vi "Get Channel Array Offset.vi"(0 "private data":T1={"instruction target"=refnum, "channels"=[], "measure state"=enum."Uninitialized", "rx output divider"=enum."1", "equalization mode"=enum."DFE", "rx internal data width"=enum."32 Bit", "BER floor"=0.0, "number of points completed"=0, "rx output divider configured?"=FALSE, "equalization mode configured?"=FALSE, "rx data width configured?"=FALSE}, 5 "instance":u8, 11 "error in":errorcluster) -> (4 "private data out":T1={"instruction target"=refnum, "channels"=[], "measure state"=enum."Uninitialized", "rx output divider"=enum."1", "equalization mode"=enum."DFE", "rx internal data width"=enum."32 Bit", "BER floor"=0.0, "number of points completed"=0, "rx output divider configured?"=FALSE, "equalization mode configured?"=FALSE, "rx data width configured?"=FALSE}, 6 "channel array offset":i32, 15 "error out":errorcluster)   [LabVIEW 2015, in "niHighSpeedSerial Eye Scan v1 Host.lvclass"]
doc: "Returns the offset in the channels array of the specified instance number\n\n<B>Input Parameters</B>\n\n<B>private data</B> is the class private data input into the VI.\n\n<B>private data.instruction target</B> is the instruction target to use when communicating with the FPGA.\n\n<B>private data.channels</B> is the array of channel information.\n\n<B>private data.channels.instance</B> is the instance of the channel.\n\n<B>private data.channels.channel</B> is the channel object for a particular channel instance.\n\n<B>private data.channels.point iterator</B> is the point iterator which stores the channel's measured points and controls which point to measure next.\n\n<B>private data.measure state</B> maintains the internal state of the Eye Scan class.\nenum values: Uninitialized,Initialized,Ready,Measuring,Finished,Aborted\n\n<B>private data.rx output divider</B> represents the configuration of the receiver output divider. This should match the values configured with RXRATE and RXOUT_DIV.\nenum values: 1,2,4,8,16\n\n<B>private data.equalization mode</B> indicates the Equalization Mode that the lane is using.\nenum values: DFE,LPM\n\n<B>private data.data width</B> is the data width (in bits) of the receiver lane.\nenum values: 16 Bit,20 Bit,32 Bit,40 Bit\n\n<B>private data.BER floor</B> is the minimum Bit Error Rate which may be computed.\n\n<B>private data.number of points completed</B> is the number of points that have been completed so far by Eye Scan.\n\n<B>private data.rx output divider configured?</B> is true if you have configured the RX Output Divider.\n\n<B>private data.equalization mode configured?</B> is true if you have configured the Equalization Mode\n\n<B>private data.data width configured?</B> is true if you have configured the Data Width.\n\n<B>instance</B> The instance of the channel to be used.\n\n<B>error in</B> describes error conditions that occur before this node runs. This input provides standard 'error in' functionality.\n\n<B>Output Parameters</B>\n\n<B>private data out</B> is the class private data output from the VI.\n\n<B>private data out.instruction target</B> is the instruction target to use when communicating with the FPGA.\n\n<B>private data out.channels</B> is the array of channel information.\n\n<B>private data out.channels.instance</B> is the instance of the channel.\n\n<B>private data out.channels.channel</B> is the channel object for a particular channel instance.\n\n<B>private data out.channels.point iterator</B> is the point iterator which stores the channel's measured points and controls which point to measure next.\n\n<B>private data out.measure state</B> maintains the internal state of the Eye Scan class.\nenum values: Uninitialized,Initialized,Ready,Measuring,Finished,Aborted\n\n<B>private data out.rx output divider</B> represents the configuration of the receiver output divider. This should match the values configured with RXRATE and RXOUT_DIV.\nenum values: 1,2,4,8,16\n\n<B>private data out.equalization mode</B> indicates the Equalization Mode that the lane is using.\nenum values: DFE,LPM\n\n<B>private data out.data width</B> is the data width (in bits) of the receiver lane.\nenum values: 16 Bit,20 Bit,32 Bit,40 Bit\n\n<B>private data out.BER floor</B> is the minimum Bit Error Rate which may be computed.\n\n<B>private data out.number of points completed</B> is the number of points that have been completed so far by the Eye Scan algorithm.\n\n<B>private data out.rx output divider configured?</B> is true if you have configured the RX Output Divider.\n\n<B>private data out.equalization mode configured?</B> is true if you have configured the Equalization Mode.\n\n<B>private data out.data width configured?</B> is true if you have configured the Data Width.\n\n<B>channel array offset</B> is the offset of the channel represented by the passed in instance number.\n\n<B>error out</B> contains error information. This output provides standard 'error out' functionality."
uses:
  <instrlib>/niHighSpeedSerial/Eye Scan/v1/Host/Eye Scan/niHighSpeedSerial Eye Scan v1 Host.lvclass
  <instrlib>/niHighSpeedSerial/Eye Scan/v1/Host/Eye Scan/Private/Private Data.ctl
  <instrlib>/_niInstr/Instruction Framework/v1/Host/Instruction Target/niInstr Instruction Target v1 Host.lvclass
  <instrlib>/niHighSpeedSerial/Eye Scan/v1/Host/Eye Scan/Private/Channel Data.ctl
  <instrlib>/niHighSpeedSerial/Eye Scan/v1/Host/Impl/Single Point/niHighSpeedSerial Eye Scan Single Point v1 Host.lvclass
  <instrlib>/niHighSpeedSerial/Eye Scan/v1/Host/Impl/Eye Scan Point Iterator/niHighSpeedSerial Eye Scan Point Iterator v1 Host.lvclass
  <instrlib>/niHighSpeedSerial/Eye Scan/v1/Host/Eye Scan/Private/Measure State.ctl
  <instrlib>/niHighSpeedSerial/Eye Scan/v1/Host/Common/Public/RX Output Divider.ctl
  <instrlib>/niHighSpeedSerial/Eye Scan/v1/Host/Common/Public/Equalization Mode.ctl
  <instrlib>/niHighSpeedSerial/Eye Scan/v1/Host/Common/Public/Data Width.ctl
  <vilib>/Utility/error.llb/Error Cluster From Error Code.vi
  <vilib>/ErrorRing/Error Ring.xnode
  <instrlib>/niHighSpeedSerial/Eye Scan/v1/Host/Common/niHighSpeedSerial Eye Scan Common v1 Host.lvlib
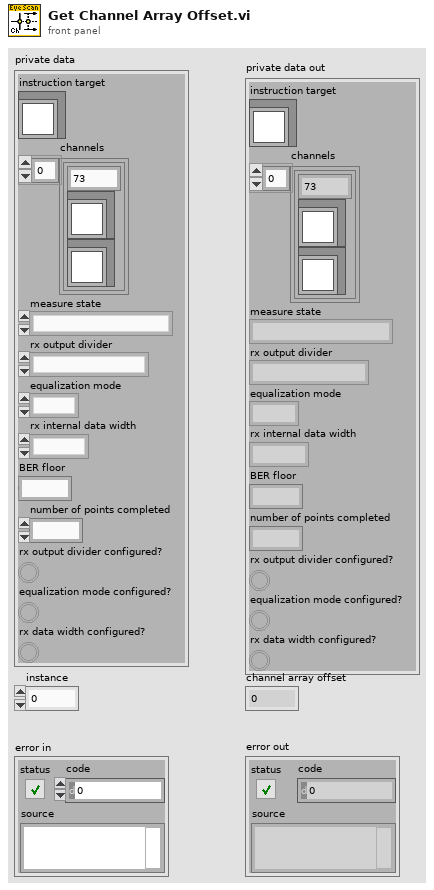
[diagram p1: front panel]
types:
  T1 = typedef "niHighSpeedSerial Eye Scan v1 Host.lvclass/Private Data.ctl" = cluster{"instruction target":refnum<class "niInstr Instruction Target v1 Host.lvclass">, "channels":T2[], "measure state":T3, "rx output divider":T4, "equalization mode":T5, "rx internal data width":T6, "BER floor":dbl, "number of points completed":i32, "rx output divider configured?":bool, "equalization mode configured?":bool, "rx data width configured?":bool}
  T2 = typedef "niHighSpeedSerial Eye Scan v1 Host.lvclass/Channel Data.ctl" = cluster{"instance":u8, "channel":refnum<class "niHighSpeedSerial Eye Scan Single Point v1 Host.lvclass">, "point iterator":refnum<class "niHighSpeedSerial Eye Scan Point Iterator v1 Host.lvclass">}
  T3 = typedef "niHighSpeedSerial Eye Scan v1 Host.lvclass/Measure State.ctl" = enum16{"Uninitialized", "Initialized", "Ready", "Measuring", "Finished", "Aborted"}
  T4 = typedef "niHighSpeedSerial Eye Scan Common v1 Host.lvlib/RX Output Divider.ctl" = enum16{"1", "2", "4", "8", "16"}
  T5 = typedef "niHighSpeedSerial Eye Scan Common v1 Host.lvlib/Equalization Mode.ctl" = enum16{"DFE", "LPM"}
  T6 = typedef "niHighSpeedSerial Eye Scan Common v1 Host.lvlib/Data Width.ctl" = enum16{"16 Bit", "20 Bit", "32 Bit", "40 Bit"}
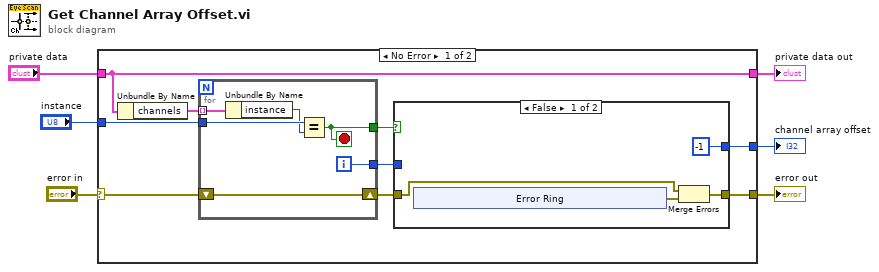
[diagram p0: block diagram]
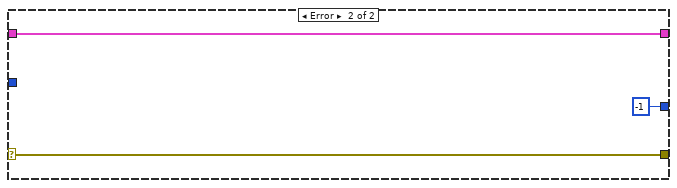
[diagram p3: hidden frame]
diagram:
  n1 = case shown="No Error" "error in" {
    selector: "error in" -> [w14 w34]
    tunnel: [w10 w34] -> w5
    tunnel: [w13 w33] -> w4
    tunnel: "private data" -> [w13 w33]
    tunnel: "instance" -> [w15 _]
    tunnel: [w7 -1] -> w1
    frame No Error {
      n2 = Unbundle By Name(w13) -> ("channels"=w12:T2[])
      n3 = for {
        tunnel: w12 -> [w31] mode=indexing
        tunnel: w15 -> [w30]
        shift-right: [w29] -> w9
        shift-left: w14 -> [w29]
        tunnel: [w28] -> w11
        tunnel: [w27] -> w8
        i -> [w27]
        stop <- w28 stop-if-true
        n4 = Unbundle By Name(w31) -> ("instance"=w26:u8)
        n5 = Equal?(x=w30, y=w26) -> (x = y?=w28:bool)
      }
      n6 = case shown="False" w11 {
        tunnel: [w18 w25] -> w10
        tunnel: w9 -> [w19 w25]
        tunnel: [-1 w24] -> w7
        tunnel: w8 -> [_ w24]
        frame False {
          n7 = xnode "Error Ring"() -> ("error out"=w16:errorcluster)
          n8 = Merge Errors(w19, w16) -> (w18:errorcluster)
        }
        frame True {
        }
      }
    }
    frame Error {
    }
  }
  "error out" <- w5
  "private data out" <- w4
  "channel array offset" <- w1
